vi "Home Page.vi"() -> (4 "Home Msg":string="    Parameters for measuring ADC: \n\n            1. DNL  \n\n            2. INL  \n\n \nDNL:\n\n   * Differential Non-Linearity (DNL) is the difference between two successive voltage levels that the DAC produces. \n\n   * Difference between the actual step width occurred and ideal step width for the corresponding voltage. \n\n   * The ideal difference between two successive voltages is 1 LSB. \n\n   * To generate DNL, take the difference of  Vout value from one transition to the next transition and ideal value. \n\nINL:\n\n   * Integral Non-Linearity (INL) is the maximum deviation of actual input-output characteristics from the ideal transfer characteristics. \n\n   * It is measured by using the Endpoint method. \n\n   * If the INL of a DAC is less than ±0.5 LSb, the input-output characteristic is monotonic.  ")   [LabVIEW 2020, in "INL DNL Test.lvclass"]
uses:
  INL DNL Test.lvclass
  Typedef/User event controls.ctl
  INL DNL Test.lvclass/INL DNL Test.ctl
  DNL INL Test.lvlib
panel:
  out "Error Out":errorcluster
  in  "Error In":errorcluster
  # "DNL and INL Test"
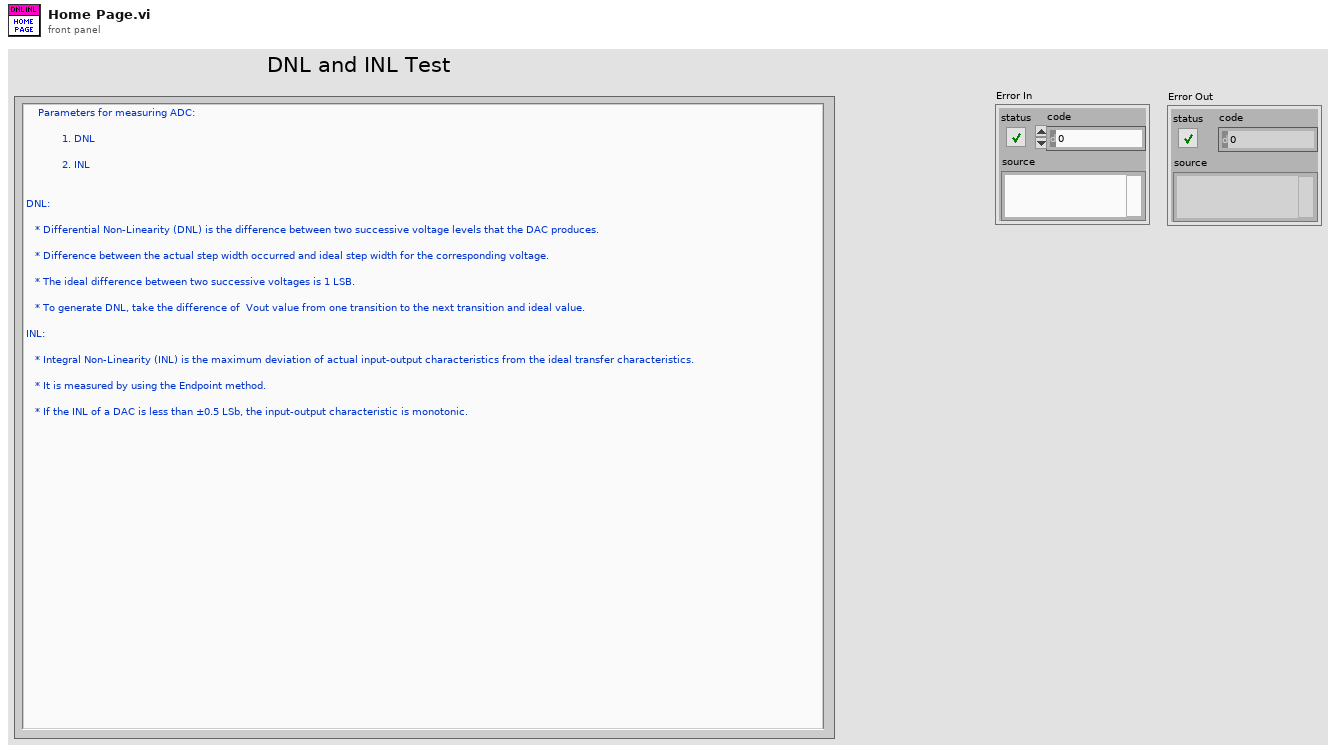
[diagram p1: front panel]
types:
  T1 = typedef "DNL INL Test.lvlib/User event controls.ctl" = enum16{"Create", "Generate", "Run Test", "Get Ref", "Destroy"}
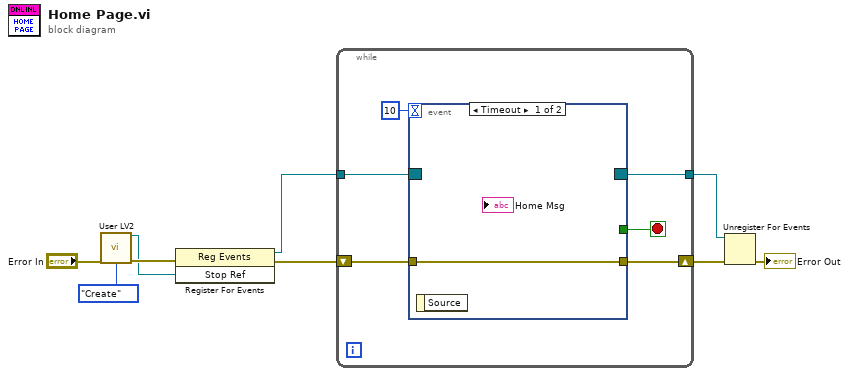
[diagram p0: block diagram]
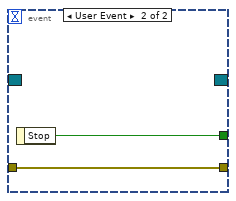
[diagram p2: hidden frame]
diagram:
  n1 = call "User LV2.vi"("Error In"="Error In", "User event controls"=User_event_controls."Create") -> ("Stop Ref"=w5:refnum<user-event>, "Error Out"=w7:errorcluster)  [unwired: 11 in, 1 out]
  n2 = register-events(error in=w7, w5) -> (reference out=w9:refnum<event-registration>, error out=w4:errorcluster)  [unwired: 1 in]
  n3 = while {
    tunnel: w9 -> [w15]
    tunnel: [w13] -> w2
    shift-right: [w11] -> w3
    shift-left: w4 -> [w12]
    stop <- w14 stop-if-true
    n4 = event shown="[0] Timeout" {
      selector: w15 -> [_ _]
      dyn-events: [_ _] -> w13
      timeout: 10 -> [_ _]
      tunnel: [_ w18] -> w14
      tunnel: [w16 w17] -> w11
      tunnel: w12 -> [w16 w17]
      event Timeout {
        n5 = event-data() -> ()  [unwired: 1 in, 1 out]
      }
      event User Event {
        n6 = event-data() -> ("Stop"=w18:bool)  [unwired: 1 in]
      }
    }
  }
  n7 = Unregister For Events(event registration refnum=w2, error in=w3) -> (error out=→"Error Out":errorcluster)
